vi "punto #2.vi"() -> ()   [LabVIEW 2019]
panel:
  out "tanque vacio":bool
  out "tanque lleno":bool
  in  "llenado/vaciado":bool
  in  "accion":bool
  in  "velocidad":bool
  out "paro":bool
  out "llenando":bool
  out "vaciando":bool
  out "Tank":dbl(slide) scale=0.0..1000.0
  # "llenar"
  # "alta"
  # "vaciar"
  # "baja"
  # "continuar"
  # "parar"
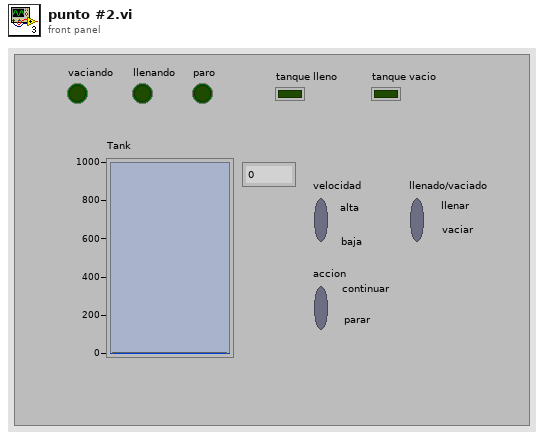
[diagram p1: front panel]
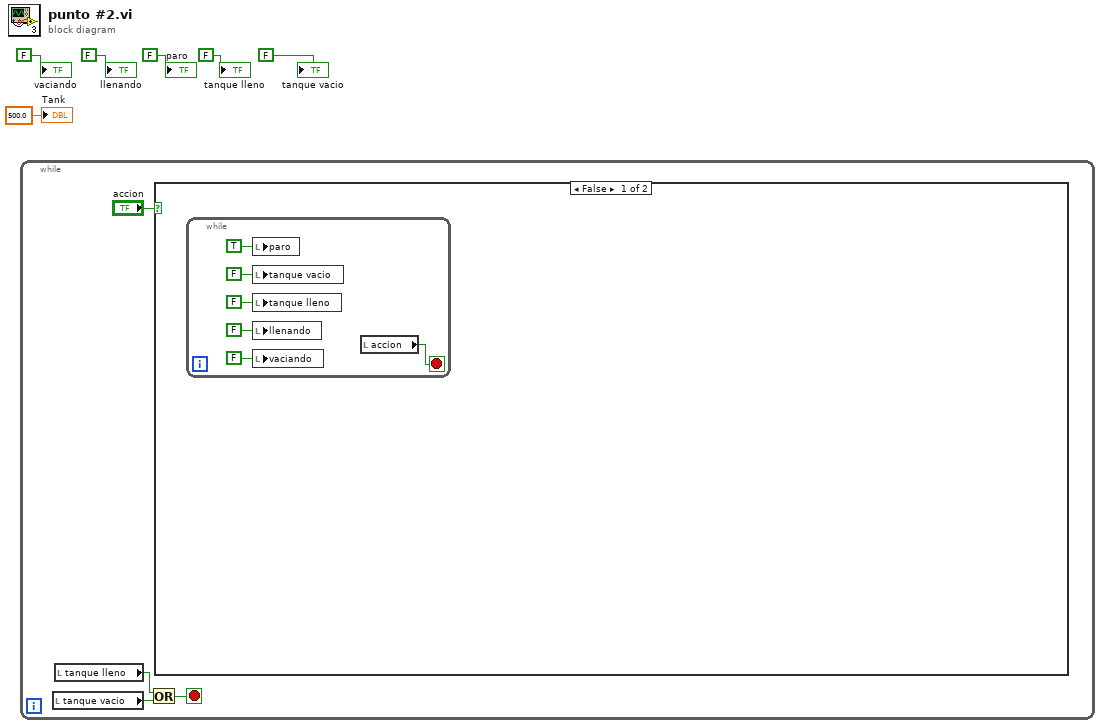
[diagram p0: block diagram]
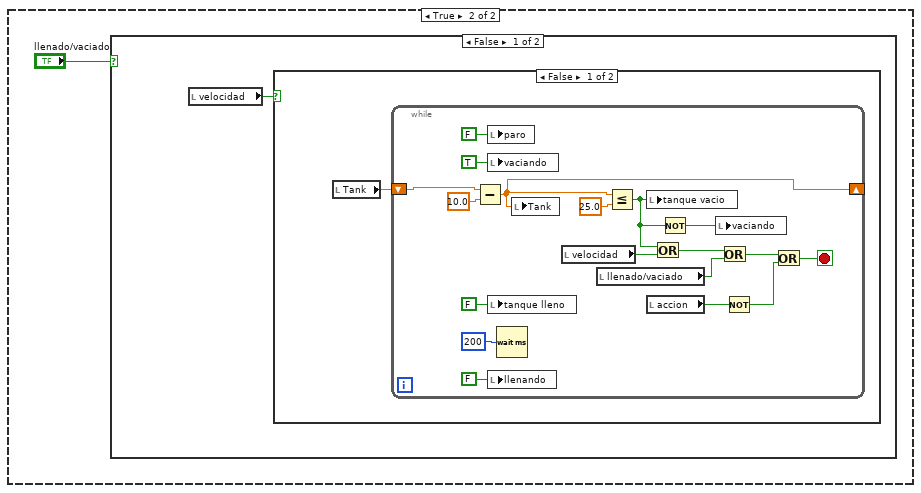
[diagram p2: hidden frame]
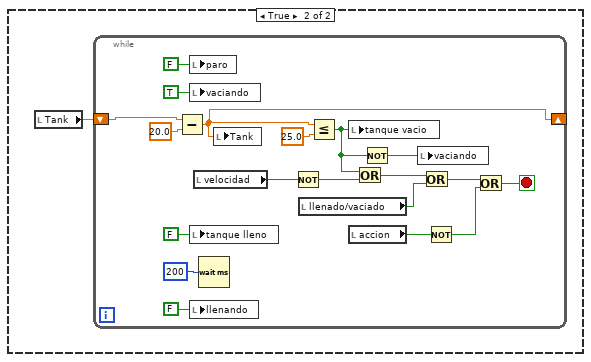
[diagram p3: hidden frame]
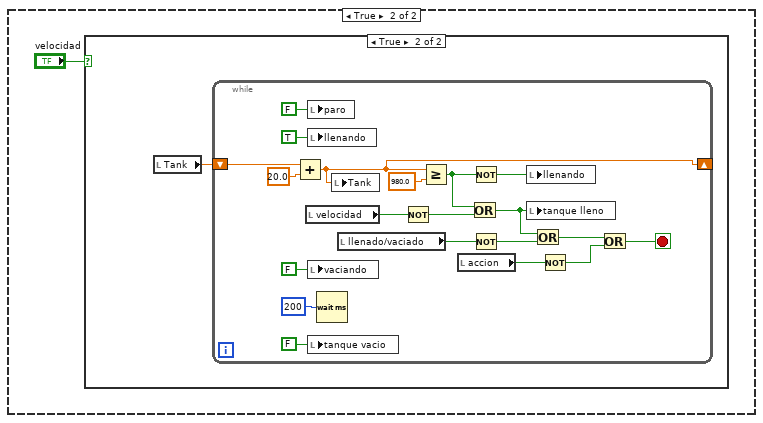
[diagram p4: hidden frame]
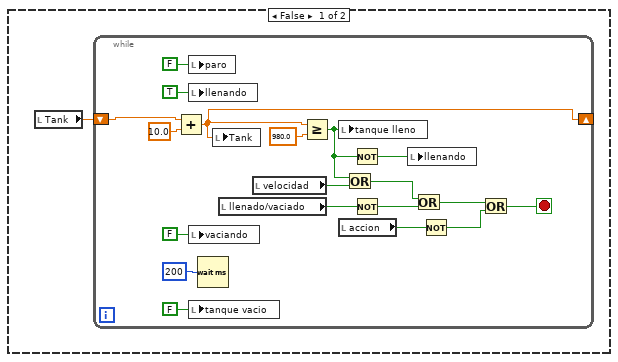
[diagram p5: hidden frame]
diagram:
  n1 = while {
    stop <- w9 stop-if-true
    n2 = local read "tanque vacio"() -> (w7:bool)
    n3 = local read "tanque lleno"() -> (w8:bool)
    n4 = Or(x=w8, y=w7) -> (x .or. y?=w9:bool)
    n5 = case shown="False" "accion" {
      frame False {
        n6 = while {
          stop <- w16 stop-if-true
          n7 = local write "paro"(TRUE ("paro")) -> ()
          n8 = local write "tanque vacio"(FALSE ("tanque vacio")) -> ()
          n9 = local write "tanque lleno"(FALSE ("tanque lleno")) -> ()
          n10 = local write "llenando"(FALSE ("llenando")) -> ()
          n11 = local write "vaciando"(FALSE ("vaciando")) -> ()
          n12 = local read "accion"() -> (w16:bool)
        }
      }
      frame True {
        n13 = case shown="False" "llenado/vaciado" {
          frame False {
            n14 = local read "velocidad"() -> (w18:bool)
            n15 = case shown="False" w18 {
              frame False {
                n16 = local read "Tank"() -> (w19:dbl)
                n17 = while {
                  shift-right: [w35] -> _
                  shift-left: w19 -> [w37]
                  stop <- w20 stop-if-true
                  n18 = Subtract(x=w37, y=10.0) -> (x-y=w35:dbl)
                  n19 = local write "paro"(FALSE ("paro")) -> ()
                  n20 = local write "vaciando"(TRUE ("vaciando")) -> ()
                  n21 = local write "tanque lleno"(FALSE ("tanque lleno")) -> ()
                  n22 = local write "llenando"(FALSE ("llenando")) -> ()
                  n23 = Wait (ms)(milliseconds to wait=u32 200) -> ()  [unwired: 1 out]
                  n24 = local write "Tank"(w35) -> ()
                  n25 = local read "velocidad"() -> (w32:bool)
                  n26 = local read "llenado/vaciado"() -> (w30:bool)
                  n27 = Less Or Equal?(x=w35, y=25.0) -> (x <= y?=w28:bool)
                  n28 = local write "tanque vacio"(w28) -> ()
                  n29 = local read "accion"() -> (w25:bool)
                  n30 = Or(x=w28, y=w32) -> (x .or. y?=w31:bool)
                  n31 = Not(x=w28) -> (.not. x?=w27:bool)
                  n32 = local write "vaciando"(w27) -> ()
                  n33 = Or(x=w31, y=w30) -> (x .or. y?=w22:bool)
                  n34 = Not(x=w25) -> (.not. x?=w29:bool)
                  n35 = Or(x=w22, y=w29) -> (x .or. y?=w20:bool)
                }
              }
              frame True {
                n36 = local read "Tank"() -> (w38:dbl)
                n37 = while {
                  shift-right: [w56] -> _
                  shift-left: w38 -> [w57]
                  stop <- w46 stop-if-true
                  n38 = Subtract(x=w57, y=20.0) -> (x-y=w56:dbl)
                  n39 = local write "paro"(FALSE ("paro")) -> ()
                  n40 = local write "vaciando"(TRUE ("vaciando")) -> ()
                  n41 = local write "tanque lleno"(FALSE ("tanque lleno")) -> ()
                  n42 = local write "llenando"(FALSE ("llenando")) -> ()
                  n43 = local read "velocidad"() -> (w51:bool)
                  n44 = Wait (ms)(milliseconds to wait=u32 200) -> ()  [unwired: 1 out]
                  n45 = local write "Tank"(w56) -> ()
                  n46 = Not(x=w51) -> (.not. x?=w50:bool)
                  n47 = local read "llenado/vaciado"() -> (w49:bool)
                  n48 = Less Or Equal?(x=w56, y=25.0) -> (x <= y?=w44:bool)
                  n49 = local write "tanque vacio"(w44) -> ()
                  n50 = local read "accion"() -> (w52:bool)
                  n51 = Or(x=w44, y=w50) -> (x .or. y?=w45:bool)
                  n52 = Not(x=w44) -> (.not. x?=w40:bool)
                  n53 = local write "vaciando"(w40) -> ()
                  n54 = Or(x=w45, y=w49) -> (x .or. y?=w47:bool)
                  n55 = Not(x=w52) -> (.not. x?=w48:bool)
                  n56 = Or(x=w47, y=w48) -> (x .or. y?=w46:bool)
                }
              }
            }
          }
          frame True {
            n57 = case shown="True" "velocidad" {
              frame False {
                n58 = local read "Tank"() -> (w59:dbl)
                n59 = while {
                  shift-right: [w77] -> _
                  shift-left: w59 -> [w78]
                  stop <- w65 stop-if-true
                  n60 = Add(x=w78, y=10.0) -> (x+y=w77:dbl)
                  n61 = local write "paro"(FALSE ("paro")) -> ()
                  n62 = local write "llenando"(TRUE ("llenando")) -> ()
                  n63 = local write "vaciando"(FALSE ("vaciando")) -> ()
                  n64 = local write "tanque vacio"(FALSE ("tanque vacio")) -> ()
                  n65 = Wait (ms)(milliseconds to wait=u32 200) -> ()  [unwired: 1 out]
                  n66 = local write "Tank"(w77) -> ()
                  n67 = local read "llenado/vaciado"() -> (w73:bool)
                  n68 = local read "velocidad"() -> (w71:bool)
                  n69 = Greater Or Equal?(x=w77, y=980.0) -> (x >= y?=w70:bool)
                  n70 = local write "tanque lleno"(w70) -> ()
                  n71 = local read "accion"() -> (w72:bool)
                  n72 = Or(x=w70, y=w71) -> (x .or. y?=w68:bool)
                  n73 = Not(x=w70) -> (.not. x?=w69:bool)
                  n74 = Not(x=w73) -> (.not. x?=w67:bool)
                  n75 = local write "llenando"(w69) -> ()
                  n76 = Or(x=w68, y=w67) -> (x .or. y?=w61:bool)
                  n77 = Not(x=w72) -> (.not. x?=w66:bool)
                  n78 = Or(x=w61, y=w66) -> (x .or. y?=w65:bool)
                }
              }
              frame True {
                n79 = local read "Tank"() -> (w79:dbl)
                n80 = while {
                  shift-right: [w98] -> _
                  shift-left: w79 -> [w99]
                  stop <- w88 stop-if-true
                  n81 = Add(x=w99, y=20.0) -> (x+y=w98:dbl)
                  n82 = local read "velocidad"() -> (w83:bool)
                  n83 = local write "paro"(FALSE ("paro")) -> ()
                  n84 = local write "llenando"(TRUE ("llenando")) -> ()
                  n85 = local write "vaciando"(FALSE ("vaciando")) -> ()
                  n86 = local write "tanque vacio"(FALSE ("tanque vacio")) -> ()
                  n87 = Wait (ms)(milliseconds to wait=u32 200) -> ()  [unwired: 1 out]
                  n88 = local write "Tank"(w98) -> ()
                  n89 = local read "llenado/vaciado"() -> (w92:bool)
                  n90 = Not(x=w83) -> (.not. x?=w94:bool)
                  n91 = Greater Or Equal?(x=w98, y=980.0) -> (x >= y?=w85:bool)
                  n92 = local read "accion"() -> (w91:bool)
                  n93 = Or(x=w85, y=w94) -> (x .or. y?=w87:bool)
                  n94 = Not(x=w85) -> (.not. x?=w81:bool)
                  n95 = Not(x=w92) -> (.not. x?=w93:bool)
                  n96 = local write "llenando"(w81) -> ()
                  n97 = local write "tanque lleno"(w87) -> ()
                  n98 = Or(x=w87, y=w93) -> (x .or. y?=w89:bool)
                  n99 = Not(x=w91) -> (.not. x?=w90:bool)
                  n100 = Or(x=w89, y=w90) -> (x .or. y?=w88:bool)
                }
              }
            }
          }
        }
      }
    }
  }
  "Tank" <- 500.0 ("Tank")
  "vaciando" <- FALSE ("vaciando")
  "llenando" <- FALSE ("llenando")
  "paro" <- FALSE ("paro")
  "tanque lleno" <- FALSE ("tanque lleno")
  "tanque vacio" <- FALSE ("tanque vacio")
